vi "Quote String.vi"(10 "String In":string) -> (2 "Quoted String":string)   [LabVIEW 2014, in "Robot Actor Framework.lvlib" / "Trace.lvlib" / "Trace.lvclass"]
uses:
  Trace.lvclass
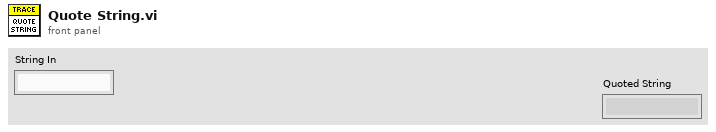
[diagram p1: front panel]
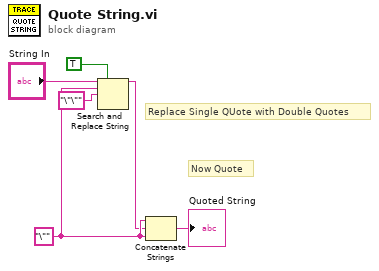
[diagram p0: block diagram]
diagram:
  w4 = "\"" ("string")
  # "Now Quote"
  # "Replace Single QUote with Double Quotes"
  n1 = Search and Replace String(replace all?=TRUE ("replace all? (F)"), input string="String In", search string=w4, replace string="\"\"" ("replace string (\"\")")) -> (result string=w2:string)  [unwired: 4 in, 3 out]
  n2 = Concatenate Strings(w4, w2, w4) -> (→"Quoted String":string)
